vi "convertChannelNames.vi"(8 "error in (no error)":errorcluster, 10 "physicalChannels":string, 11 "K2602 in":refnum<class "K2602.lvclass">) -> (0 "error out":errorcluster, 2 "channels":string[](array[string]), 3 "K2602 out":refnum<class "K2602.lvclass">)   [LabVIEW 2011, in "Hardware.lvlib" / "Channels.lvlib" / "K2602.lvclass"]
uses:
  K2602.lvclass
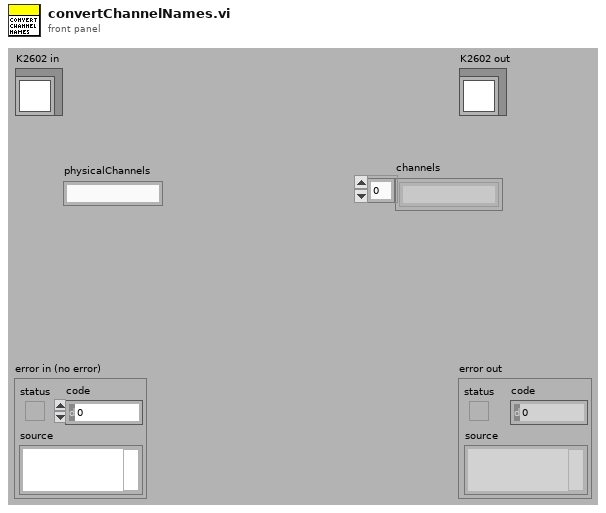
[diagram p1: front panel]
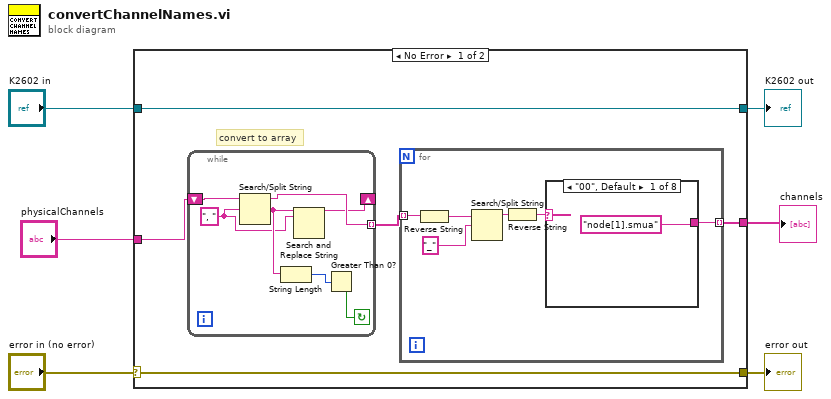
[diagram p0: block diagram]
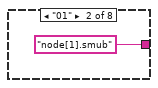
[diagram p2: hidden frame]
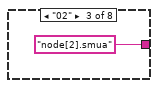
[diagram p3: hidden frame]
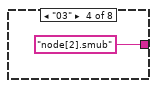
[diagram p4: hidden frame]
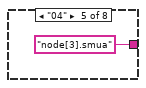
[diagram p5: hidden frame]
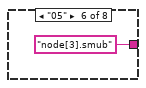
[diagram p6: hidden frame]
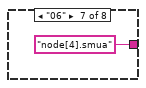
[diagram p7: hidden frame]
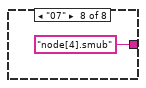
[diagram p8: hidden frame]
diagram:
  n1 = case shown="No Error" "error in (no error)" {
    selector: "error in (no error)" -> [w10 w34]
    tunnel: [w10 w34] -> w5
    tunnel: [w11 w33] -> w3
    tunnel: "K2602 in" -> [w11 w33]
    tunnel: "physicalChannels" -> [w9 _]
    tunnel: [w7 _] -> w1
    frame No Error {
      # "convert to array"
      n2 = while {
        shift-right: [w26] -> _
        shift-left: w9 -> [w27]
        tunnel: [w32] -> w8 mode=indexing
        stop <- w28 continue-if-true
        w30 = ", "
        n3 = Search/Split String(string=w27, search string/char (-)=w30) -> (substring before match=w32:string, match + rest of string=w31:string)  [unwired: 1 in, 1 out]
        n4 = String Length(string=w31) -> (length=w29:i32)
        n5 = Search and Replace String(input string=w31, search string=w30) -> (result string=w26:string)  [unwired: 6 in, 3 out]
        n6 = Greater Than 0?(x=w29) -> (x > 0?=w28:bool)
      }
      n7 = for {
        tunnel: w8 -> [w17] mode=indexing
        tunnel: [w12] -> w7 mode=indexing
        n8 = Reverse String(1:w17) -> (0:w16:string)
        n9 = Search/Split String(string=w16, search string/char (-)="_") -> (substring before match=w14:string)  [unwired: 1 in, 2 out]
        n10 = Reverse String(1:w14) -> (0:w13:string)
        n11 = case shown="\"00\", Default" w13 {
          tunnel: ["node[1].smua" "node[1].smub" "node[2].smua" "node[2].smub" "node[3].smua" "node[3].smub" "node[4].smua" "node[4].smub"] -> w12
          frame "00", Default {
          }
          frame "01" {
          }
          frame "02" {
          }
          frame "03" {
          }
          frame "04" {
          }
          frame "05" {
          }
          frame "06" {
          }
          frame "07" {
          }
        }
      }
    }
    frame Error {
    }
  }
  "error out" <- w5
  "K2602 out" <- w3
  "channels" <- w1
